vi "decode_posit_rs16.vi"(4 "x":i16) -> (0 "rs":i16, 1 "reg":i16)   [LabVIEW 2018, in "posit.lvlib"]
uses:
  posit.lvlib
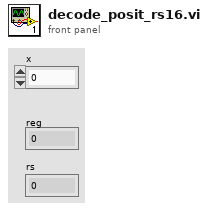
[diagram p1: front panel]
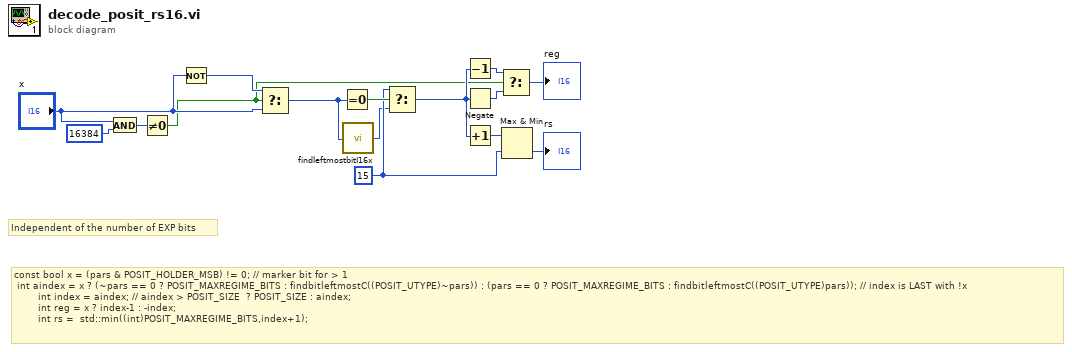
[diagram p0: block diagram]
diagram:
  w5 = i16 15 ("t")
  # "Independent of the number of EXP bits"
  # "const bool x = (pars & POSIT_HOLDER_MSB) != 0; // marker bit for > 1\n int aindex = x ? (~pars == 0 ? POSIT_MAXREGIME_BITS : findbitleftmostC((POSIT_UTYPE)~pars)) : (pars == 0 ? POSIT_MAXREGIME_BITS : findbitleftmostC((POSIT_UTYPE)pars)); // index is LAST with !x\n        int index = aindex; // aindex > POSIT_SIZE  ? POSIT_SIZE : aindex;\n        int reg = x ? index-1 : -index;\n        int rs =  std::min((int)POSIT_MAXREGIME_BITS,index+1);"
  n1 = And(x="x", y=i16 16384) -> (x .and. y?=w12:i16)
  n2 = Not Equal To 0?(x=w12) -> (x != 0?=w3:bool)
  n3 = Not(x="x") -> (.not. x?=w14:i16)
  n4 = Select(t=w14, s=w3, f="x") -> (s? t:f=w2:i16)
  n5 = Equal To 0?(x=w2) -> (x = 0?=w11:bool)
  n6 = call "findleftmostbitI16x.vi"("x"=w2) -> ("index"=w1:i16)
  n7 = Select(t=w5, s=w11, f=w1) -> (s? t:f=w4:i16)
  n8 = Decrement(x=w4) -> (x-1=w10:i16)
  n9 = Negate(x=w4) -> (-x=w9:i16)
  n10 = Increment(x=w4) -> (x+1=w7:i16)
  n11 = Select(t=w10, s=w3, f=w9) -> (s? t:f=→"reg":i16)
  n12 = Max & Min(x=w7, y=w5) -> (min(x,y)=→"rs":i16)  [unwired: 1 out]
